vi "Write ALR_index.vi"(6 "Find all":bool=TRUE, 9 "Heater":string, 10 "EnumsALR":string[](array[string]), 11 "Heater in":refnum<class "Heater.lvclass">) -> (2 "Find":bool, 3 "Heater out":refnum<class "Heater.lvclass">)   [LabVIEW 2019, in "Heating.lvlib" / "Heater.lvclass"]
uses:
  Heater.lvclass
  Heater.lvclass/Heater.ctl
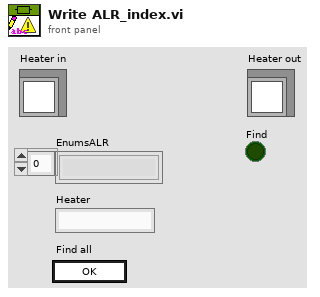
[diagram p1: front panel]
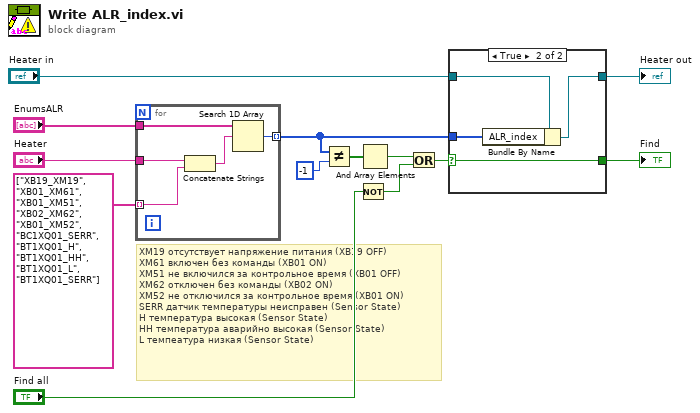
[diagram p0: block diagram]
diagram:
  # "XM19\tотсутствует напряжение питания (XB19 OFF)\nXM61\tвключен без команды (XB01 ON)\nXM51\tне включился за контрольное время (XB01 OFF)\nXM62\tотключен без команды (XB02 ON)\nXM52\tне отключился за контрольное время (XB01 ON)\nSERR датчик температуры неисправен (Sensor State)\nH температура высокая (Sensor State)\nHH температура аварийно высокая (Sensor State)\nL темпеатура низкая (Sensor State)"
  n1 = for {
    tunnel: "EnumsALR" -> [w18]
    tunnel: "Heater" -> [w17]
    tunnel: [w15] -> w13 mode=indexing
    tunnel: string[] ["XB19_XM19", "XB01_XM61", "XB01_XM51", "XB02_XM62", "XB01_XM52", "BC1XQ01_SERR", "BT1XQ01_H", "BT1XQ01_HH", "BT1XQ01_L", "BT1XQ01_SERR"] -> [w14] mode=indexing
    n2 = Concatenate Strings(w17, w14) -> (w16:string)
    n3 = Search 1D Array(1D array=w18, element=w16) -> (index of element=w15:i32)  [unwired: 1 in]
  }
  n4 = Not Equal?(x=w13, y=-1 ("index of element")) -> (x != y?=w9:bool[])
  n5 = Not(x="Find all") -> (.not. x?=w2:bool)
  n6 = And Array Elements(Boolean array=w9) -> (logical AND=w3:bool)
  n7 = Or(x=w3, y=w2) -> (x .or. y?=w4:bool)
  n8 = case shown="True" w4 {
    selector: w4 -> [_ w20]
    tunnel: [w19 w22] -> w5
    tunnel: "Heater in" -> [w19 w23]
    tunnel: w13 -> [_ w21]
    tunnel: [_ w20] -> w12
    frame False {
    }
    frame True {
      n9 = Bundle By Name(cluster=w23, "ALR_index"=w21) -> (w22:refnum<class "Heater.lvclass">)
    }
  }
  "Heater out" <- w5
  "Find" <- w12
